vi "Program_Active_Client.vi"(3 "Mode":enum16{"Program Active", "Traverse Level State"}(ring), 4 "Time till next contact (Sec)":dbl=60.0 min=0.0, 5 "Traverse level State":T1) -> ()   [LabVIEW 2020]
doc: "This is an example of using features of the VI Server as a client. It shows how you might browse from one or more applications that may be exporting data from one or more data stations. \n\nThe example shows how to query a server for its list of exported VIs, how to get references to the VIs, and how call them with the Call By Reference function."
uses:
  Sub VIs/ADAM Controls/Traverse_Level_State.ctl
  Anemometry/Anemometry Sub Vis/Globals/Meas_global.vi
  Anemometry/Anemometry Sub Vis/Globals/Preference_global.vi
  Anemometry/Anemometry Sub Vis/Globals/Dynamic_call_global.ph.vi
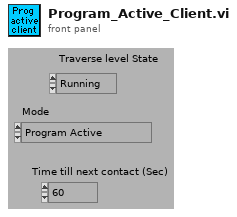
[diagram p1: front panel]
types:
  T1 = typedef "Traverse_Level_State.ctl" = enum16{"Running", "Complete"}
  T2 = typedef "Server_Comms.ctl" = enum16{"Do Not Link To Server", "Server Link Healthy"}
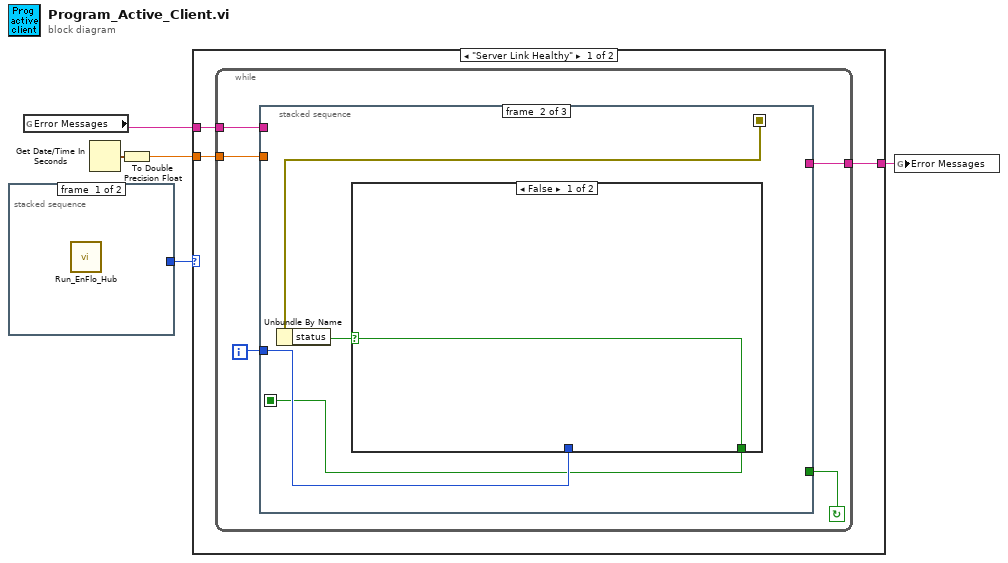
[diagram p0: block diagram]
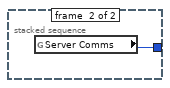
[diagram p2: hidden frame]
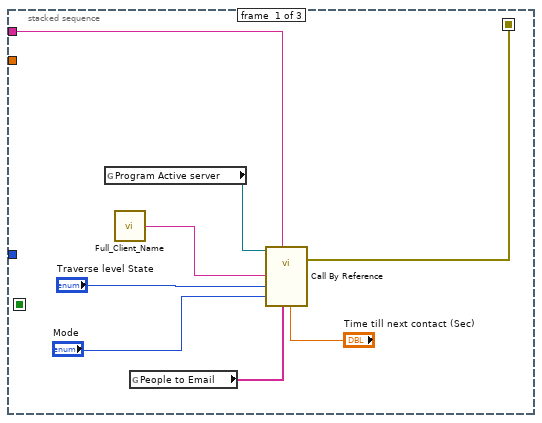
[diagram p3: hidden frame]
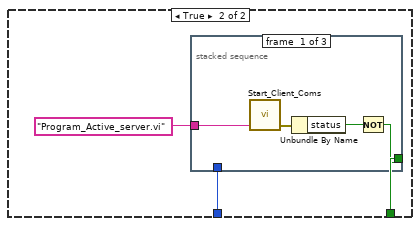
[diagram p4: hidden frame]
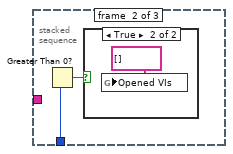
[diagram p5: hidden frame]
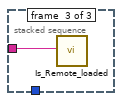
[diagram p7: hidden frame]
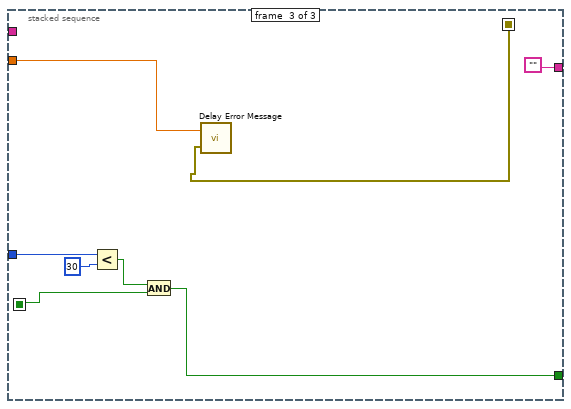
[diagram p8: hidden frame]
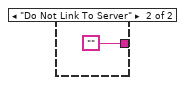
[diagram p9: hidden frame]
diagram:
  n1 = stacked-sequence {
    tunnel: [_ w6] -> w3
    frame #0 {
      n2 = call "Run_EnFlo_Hub.vi"() -> ()  [unwired: 1 in, 7 out]
    }
    frame #1 {
      n3 = global read "Preference_global.vi" "Server Comms"() -> (w6:T2)
    }
  }
  n4 = global read "Meas_global.vi" "Error Messages"() -> (w5:string)
  n5 = Get Date/Time In Seconds() -> (seconds since 1Jan1904=w2:timestamp)
  n6 = To Double Precision Float(number=w2) -> (double precision float=w1:dbl)
  n7 = case shown="\"Server Link Healthy\"" w3 {
    tunnel: w5 -> [w9 _]
    tunnel: [w8 ""] -> w4
    tunnel: w1 -> [w7 _]
    frame "Server Link Healthy" {
      n8 = while {
        tunnel: [w11] -> w8
        tunnel: w9 -> [w12]
        tunnel: w7 -> [w10]
        i -> [w14]
        stop <- w13 continue-if-true
        n9 = stacked-sequence {
          seq-local: [w22 _ _] -> [_ w25 w40]
          seq-local: [_ w23 _] -> [_ _ w43]
          tunnel: w14 -> [_ w24 w44]
          tunnel: [_ _ w42] -> w13
          tunnel: w12 -> [w17 _ _]
          tunnel: [_ _ ""] -> w11
          tunnel: w10 -> [_ _ w39]
          frame #0 {
            n10 = global read "Dynamic_call_global.ph.vi" "Program Active server"() -> (w16:refnum<vi>)
            n11 = call "Full_Client_Name.vi"() -> ("Client Name"=w18:string)
            n12 = global read "Meas_global.vi" "People to Email"() -> (w19:string[])
            n13 = call-by-ref "?"(reference=w16, "Client Name"=w18, "Client Messages"=w17, "Traverse level State"="Traverse level State", "Mode"="Mode", "People to Email"=w19, "Time till next contact (Sec)"="Time till next contact (Sec)") -> (error out=w22:errorcluster)  [unwired: 6 in, 1 out]
          }
          frame #1 {
            n14 = Unbundle By Name(w25) -> ("status"=w26:bool)
            n15 = case shown="False" w26 {
              selector: w26 -> [w27 _]
              tunnel: w24 -> [_ w30]
              tunnel: [w27 w28] -> w23
              frame False {
              }
              frame True {
                n16 = stacked-sequence {
                  tunnel: "Program_Active_server.vi" -> [w34 _ w38]
                  tunnel: w30 -> [_ w36 _]
                  tunnel: [w31 _ _] -> w28
                  frame #0 {
                    n17 = call "Start_Client_Coms.vi"("VI name to run on server"=w34) -> ("Error cluster"=w32:errorcluster)  [unwired: 1 in, 3 out]
                    n18 = Unbundle By Name(w32) -> ("status"=w33:bool)
                    n19 = Not(x=w33) -> (.not. x?=w31:bool)
                  }
                  frame #1 {
                    n20 = Greater Than 0?(x=w36) -> (x > 0?=w35:bool)
                    n21 = case shown="True" w35 {
                      frame False {
                      }
                      frame True {
                        n22 = global write "Dynamic_call_global.ph.vi" "Opened VIs"(string[] [] ("Opened VIs")) -> ()
                      }
                    }
                  }
                  frame #2 {
                    n23 = call "Is_Remote_loaded.vi"("Sub VI to call"=w38) -> ()
                  }
                }
              }
            }
          }
          frame #2 {
            n24 = Less?(x=w44, y=30) -> (x < y?=w46:bool)
            n25 = And(x=w46, y=w43) -> (x .and. y?=w42:bool)
            n26 = call "Delay Error Message.vi"("error in (no error)"=w40, "Seconds since 1904"=w39) -> ()  [unwired: 2 in]
          }
        }
      }
    }
    frame "Do Not Link To Server" {
    }
  }
  n27 = global write "Meas_global.vi" "Error Messages"(w4) -> ()
